vi "csmdoc_load vi description map.vi"(8 "Error in":errorcluster caption="Error in (no error)", 11 "Path":path=path "D:/github/JKI-State-Machine-Plus/.doc/VI Description.md") -> (0 "Error out":errorcluster, 1 "text":string, 3 "variant":variant)   [LabVIEW 2017]
uses:
  Communicable State Machine.lvlib
panel:
  out "values":string
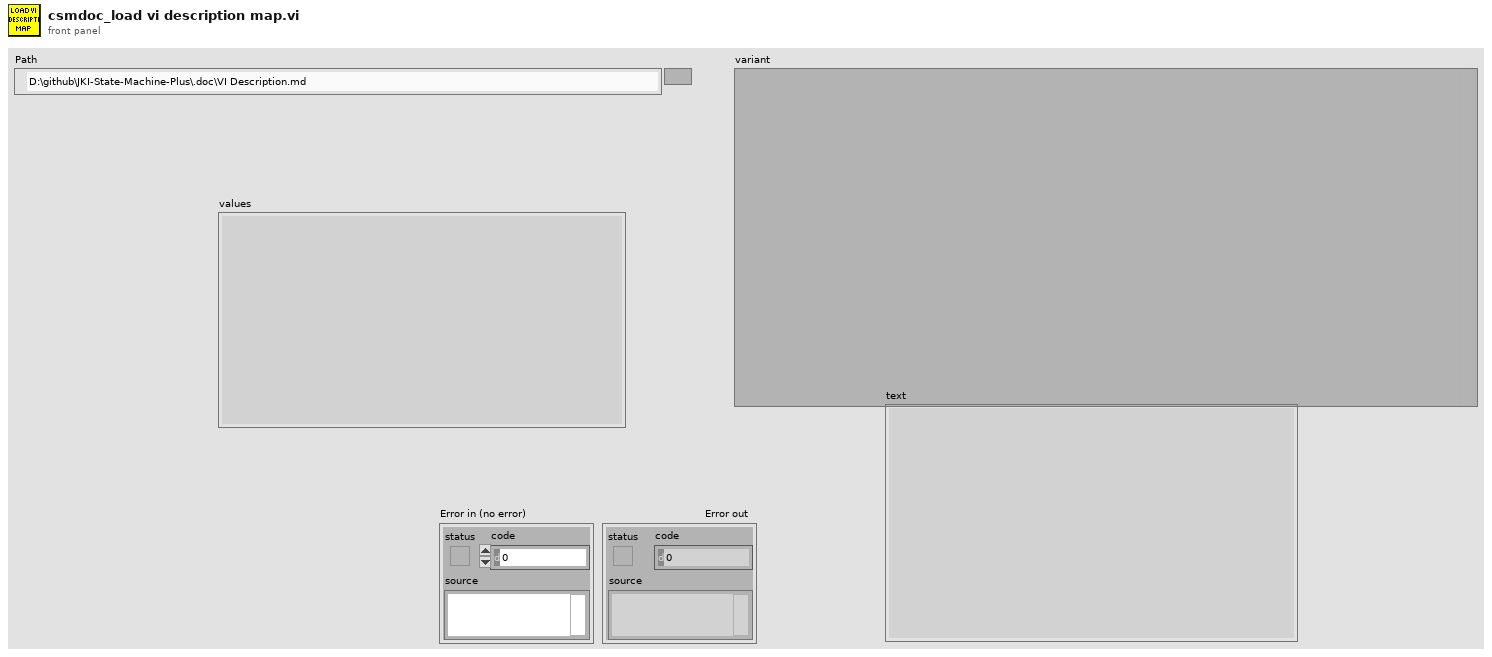
[diagram p1: front panel]
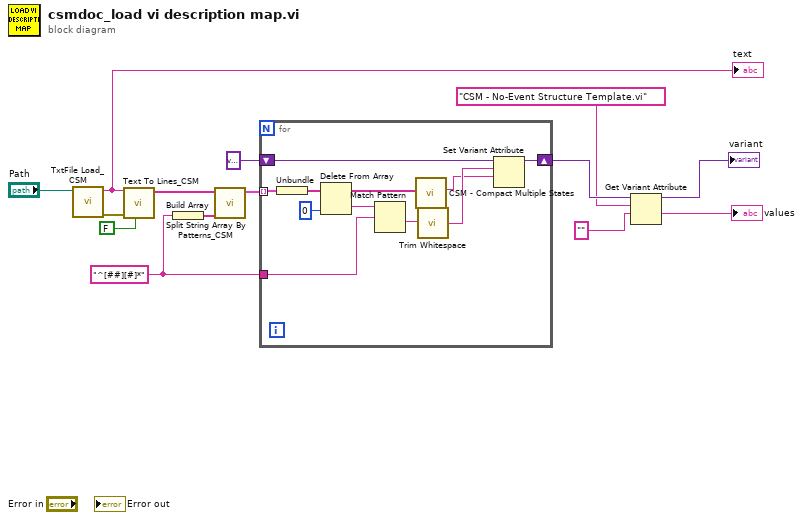
[diagram p0: block diagram]
diagram:
  w9 = "^[##][#]*" ("delimited string")
  n1 = call "TxtFile Load_CSM.vi"("Path"="Path") -> ("error out"=w13:errorcluster, "text"=w12:string)  [unwired: 9 in]
  "text" <- w12
  n2 = call "Text To Lines_CSM.vi"("Remove Empty Lines?(T)"=FALSE, "error in (no error)"=w13, "string"=w12) -> ("Lines"=w11:string[])  [unwired: 7 in, 1 out]
  n3 = Build Array(w9) -> (w8:string[])
  n4 = call "Split String Array By Patterns_CSM.vi"("patterns"=w8, "Text Array"=w11) -> ("Array"=w10:cluster{"filtered array":string[]}[])  [unwired: 9 in]
  n5 = for {
    tunnel: w10 -> [w25] mode=indexing
    tunnel: w9 -> [w21]
    shift-right: [w15] -> w5
    shift-left: variant ("variant") -> [w16]
    n6 = Unbundle(w25) -> ("filtered array"=w24:string[])
    n7 = Delete From Array(array=w24, index=0) -> (deleted portion=w22:string, array with subset deleted=w18:string[])  [unwired: 1 in]
    n8 = Match Pattern(string=w22, regular expression=w21) -> (after substring=w20:string)  [unwired: 1 in, 3 out]
    n9 = call "CSM - Compact Multiple States.vi"("Multiple States"=w18) -> ("States"=w17:string)  [unwired: 9 in]
    n10 = call <vilib>:"Trim Whitespace.vi"("string"=w20) -> ("trimmed string"=w19:string)  [unwired: 1 in]
    n11 = Set Variant Attribute(Variant=w16, name=w19, value=w17) -> (Variant out=w15:variant)  [unwired: 1 in, 2 out]
  }
  n12 = Get Variant Attribute(Variant=w5, name="CSM - No-Event Structure Template.vi", default value (empty Variant)="" ("delimited string")) -> (duplicate Variant=→"variant":variant, value=→"values":string)  [unwired: 1 in, 2 out]
